vi "Vision Processing.vi"(11 "Image In":T1) -> (3 "Height Ratio":dbl)   [LabVIEW 2017]
uses:
  <vilib>/vision/Image Controls.llb/IMAQ Image.ctl
  <vilib>/Analysis/2dsp.llb/1D Convolution (DBL).vi
  <vilib>/Analysis/NI_AALPro.lvlib
panel:
  out "error out":errorcluster
  out "Peaks":i32[](array[numeric])
  out "Index Array":i32[](array[numeric])
  out "Waveform Graph":sgl[](graph)
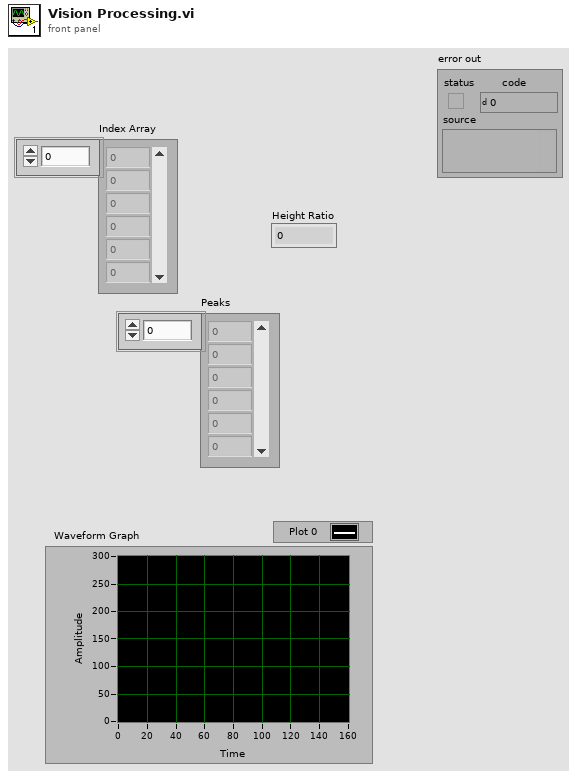
[diagram p1: front panel]
types:
  T1 = typedef "IMAQ Image.ctl" = refnum<image>
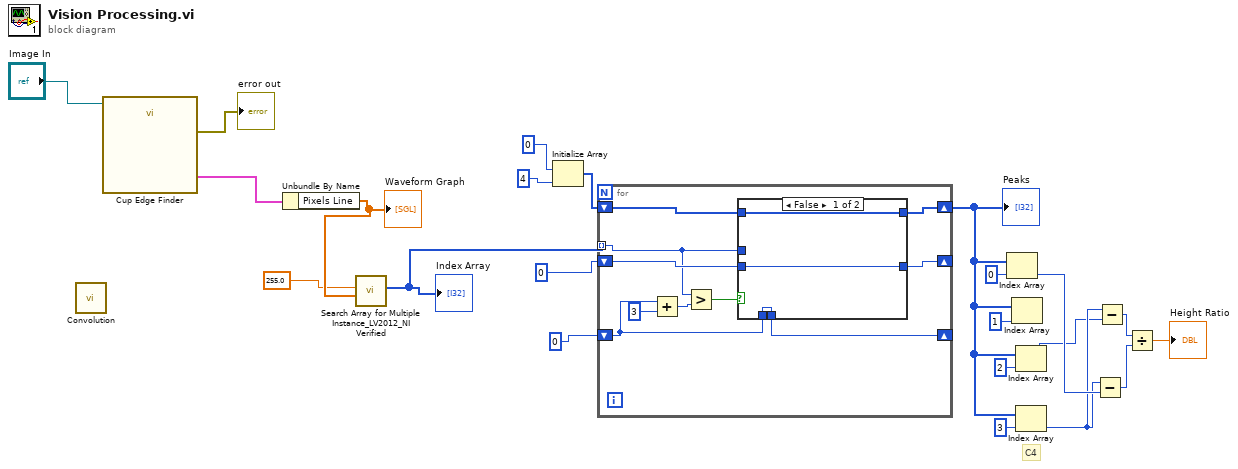
[diagram p0: block diagram]
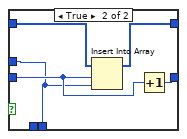
[diagram p2: hidden frame]
diagram:
  # "C4"
  n1 = call-poly <vilib>:"Convolution.vi"() -> ()  [unwired: 10 in, 2 out]
  n2 = call "Cup Edge Finder"("Image In"="Image In") -> ("Line Profile (Line Profile 1)"=w22:cluster{"x0":sgl, "dx":sgl, "Pixels Line":sgl[]}, "error out"=→"error out":errorcluster)  [unwired: 24 in, 1 out]
  n3 = Unbundle By Name(w22) -> ("Pixels Line"=w21:sgl[])
  "Waveform Graph" <- w21
  n4 = call "Search Array for Multiple Instance_LV2012_NI Verified.vi"("Array to Search"=w21, "Number to find"=255.0) -> ("Index Array"=w19:i32[])  [unwired: 9 in]
  "Index Array" <- w19
  n5 = Initialize Array(0, 4 ("dimension size")) -> (w16:i32[])
  n6 = for {
    tunnel: w19 -> [w26] mode=indexing
    shift-right: [w29] -> _
    shift-left: 0 -> [w30]
    shift-right: [w31] -> w9
    shift-left: w16 -> [w32]
    shift-right: [w28] -> _
    shift-left: 0 -> [w23]
    n7 = Add(x=w23, y=3) -> (x+y=w25:i32)
    n8 = Greater?(x=w26, y=w25) -> (0:w27:bool)
    n9 = case shown="False" w27 {
      tunnel: w32 -> [w35 w40]
      tunnel: [w35 w39] -> w31
      tunnel: w30 -> [w34 w38]
      tunnel: [w34 w37] -> w29
      tunnel: w26 -> [_ w36]
      tunnel: [w33 w36] -> w28
      tunnel: w23 -> [w33 _]
      frame False {
      }
      frame True {
        n10 = Insert Into Array(array=w40, index=w38, new element=w36) -> (w39:i32[])
        n11 = Increment(x=w38) -> (x+1=w37:i32)
      }
    }
  }
  "Peaks" <- w9
  n12 = Index Array(array=w9, index=0) -> (element=w8:i32)
  n13 = Index Array(array=w9, index=1) -> ()  [unwired: 1 out]
  n14 = Index Array(array=w9, index=2) -> (element=w2:i32)
  n15 = Index Array(array=w9, index=3) -> (element=w3:i32)
  n16 = Subtract(x=w3, y=w8) -> (x-y=w6:i32)
  n17 = Subtract(x=w3, y=w2) -> (x-y=w7:i32)
  n18 = Divide(x=w7, y=w6) -> (x/y=→"Height Ratio":dbl)
